vi "Image_Save_Handler_2.0.vi"(0 "first iteration":bool, 4 "Data":T1={"Camera 1"={"Camera1"="", "Cam 1"=FALSE, "CAM1 Model"=enum."a2A5328-15ucBAS", "Cam1 ID"=0}, "Camera 2"={"Camera2"="", "Cam 2"=FALSE, "CAM2 Model"=enum."a2A5328-15ucBAS", "Cam2 ID"=0}, "Image"={"Camera1_Img"=refnum, "Camera2_Img"=refnum, "Img1_Orig_Disp"=refnum, "Img2_Orig_Disp"=refnum, "Img1_Orig_RGB"=refnum, "Img2_Orig_RGB"=refnum, "Blue_Plane_Extract"=refnum, "Subtracted_Plane"=refnum, "Img1_Binary"=refnum, "Img2_Binary"=refnum, "Crop_Mask"=refnum, "Img1_Save"=refnum, "Img2_Save"=refnum, "Img1_Cali_Full"=refnum, "Img2_Cali_Full"=refnum, "Img1_Cali_Detect"=refnum, "Img2_Cali_Detect"=refnum}, "Ques"={"Cam 1 queue"=refnum, "Cam 2 queue"=refnum, "Cam 1 - save queue"=refnum, "Cam 2 - save queue"=refnum, "Image Process Queue Size"=500, "Image Save Queue Size"=500, "Overload threshold"=500, "Max large object threshold"=0}, "Arduino SRS"={"Pinch-valve"="", "Actuator"=FALSE, "Arduino Uno"="", "Valve state"=enum."Open"}, "Pump"={"Port"="", "Connection"=FALSE, "Flush Size"=0, "Command"="", "Pump Size"=enum."Large", "Pump"="", "Ready"=FALSE}, "Camera settings"={"Detection settings"={"Sample size threshold"=500, "Detection Region %"=30.0, "Timeout Sample"=200}, "Lens/camera settings"={"Aperture"=enum."Item 0", "Legacy Cam Attributes"=FALSE, "Max Framerate"=100, "Exposure Time"=1000.0, "Framerate"=15}, "Crop settings"={"Cam1"={"Rectangle 1"={"Left"=0, "Top"=0, "Right"=0, "Bottom"=0, "Rotation"=0.0}, "Camera Orientation 1"="", "Pixel to mm 1"=0.0}, "Cam2"={"Rectangle 2"={"Left"=0, "Top"=0, "Right"=0, "Bottom"=0, "Rotation"=0.0}, "Camera Orientation 2"="", "Pixel to mm 2"=0.0}}}, "Arduino ISS"={"Mega F3"="", "Phase3"=FALSE, "Barcode"="", "Sorting sys."=FALSE, "Initial size"=0.0, "Size Interval"=0.0, "Mun. of containers"=0.0, "Container nr."=0.0, "Arduino Mega"="", "Attempts"=0.0}, "Img_Capt"=FALSE, "Empty_Refill"=FALSE, "I don't think is in use"={"Light intensity"=100}, "Extended setup"={"Location"="Station", "Latitude"="Station", "Longitude"="Station", "Determiner"="Station", "Sex"="Station", "Station"="", "Collection date"=""}, "Main interface"={"Sample Name"="Test Sample", "Operator"="JFR", "Species Name"="", "Other Notes"=""}, "Tap1"=0, "SystemVersion"=0, "System Serial"="", "Exit"=FALSE, "Kuvette Full"=FALSE, "Core JKI"={"Current VI Reference"=refnum, "Close Panel on Exit?"=FALSE}, "Calibration"={"Calibration 1"=path "C:/Users/au540322/Desktop/IHS_Project/images/Debris/Debris_0/Debris_0_2019_06_01-23-32-49-686.PNG", "Calibration 2"=path "C:/Users/au540322/Desktop/IHS_Project/images/Debris/Debris_0/Debris_0_2019_06_01-23-32-49-686.PNG", "Detect 1"=path "C:/Users/au540322/Desktop/IHS_Project/images/Debris/Debris_0/Debris_0_2019_06_01-23-32-49-686.PNG", "Detect 2"=path "C:/Users/au540322/Desktop/IHS_Project/images/Debris/Debris_0/Debris_0_2019_06_01-23-32-49-686.PNG"}, "Auto Flush"=FALSE, "Status History"="", "Timestamp Start"=""} {"SystemVersion" items=["Standard", "XL"]; "Tap1" items=["Session Data", "Extended Setup", "Buffer", "Camera", "Dispenser", "Stats", "Connections"]; "I don't think is in use"."Light intensity" scale=0.0..100.0; "Camera settings"."Crop settings"."Cam2"."Rectangle 2"."Rotation" format="%.2f"; "Camera settings"."Crop settings"."Cam2"."Rectangle 2"."Left" scale=0.0..1024.0; "Camera settings"."Crop settings"."Cam2"."Rectangle 2"."Right" scale=0.0..1024.0; "Camera settings"."Crop settings"."Cam1"."Rectangle 1"."Rotation" format="%.2f"; "Camera settings"."Crop settings"."Cam1"."Rectangle 1"."Left" scale=0.0..1024.0; "Camera settings"."Crop settings"."Cam1"."Rectangle 1"."Right" scale=0.0..1024.0; "Camera settings"."Lens/camera settings"."Framerate" min=1; "Camera settings"."Lens/camera settings"."Max Framerate" min=1; "Camera settings"."Detection settings"."Sample size threshold" min=1; "Pump"."Flush Size" min=0 max=6000 step=100; "Ques"."Overload threshold" min=1; "Ques"."Image Save Queue Size" min=1; "Ques"."Image Process Queue Size" min=1}, 7 "Stop?":bool) -> (12 "Image Save 1":T3, 13 "Container num. Out":i32=2, 14 "Image Save 2":T3, 15 "Container barcode":string, 17 "Cam2_Stats":cluster{"Mean_Area":i32, "Img_Count":u32} caption="Camera 2", 18 "Ready file created":bool, 19 "Cam1_Stats":cluster{"Mean_Area":i32, "Img_Count":u32} caption="Camera 1", 20 "Queue size":T5, 23 "timeout":bool, 24 "max queue":i32, 25 "Sample Name":string, 27 "Stop out":bool)   [LabVIEW 2024]
doc: "Saves image files from cameras in specified folder location."
uses:
  <vilib>/vision/Image Controls.llb/IMAQ Image.ctl
  controls/Data_JKI.ctl
  <vilib>/userDefined/High Color/IMAQdx.ctl
  Camera_ID.ctl
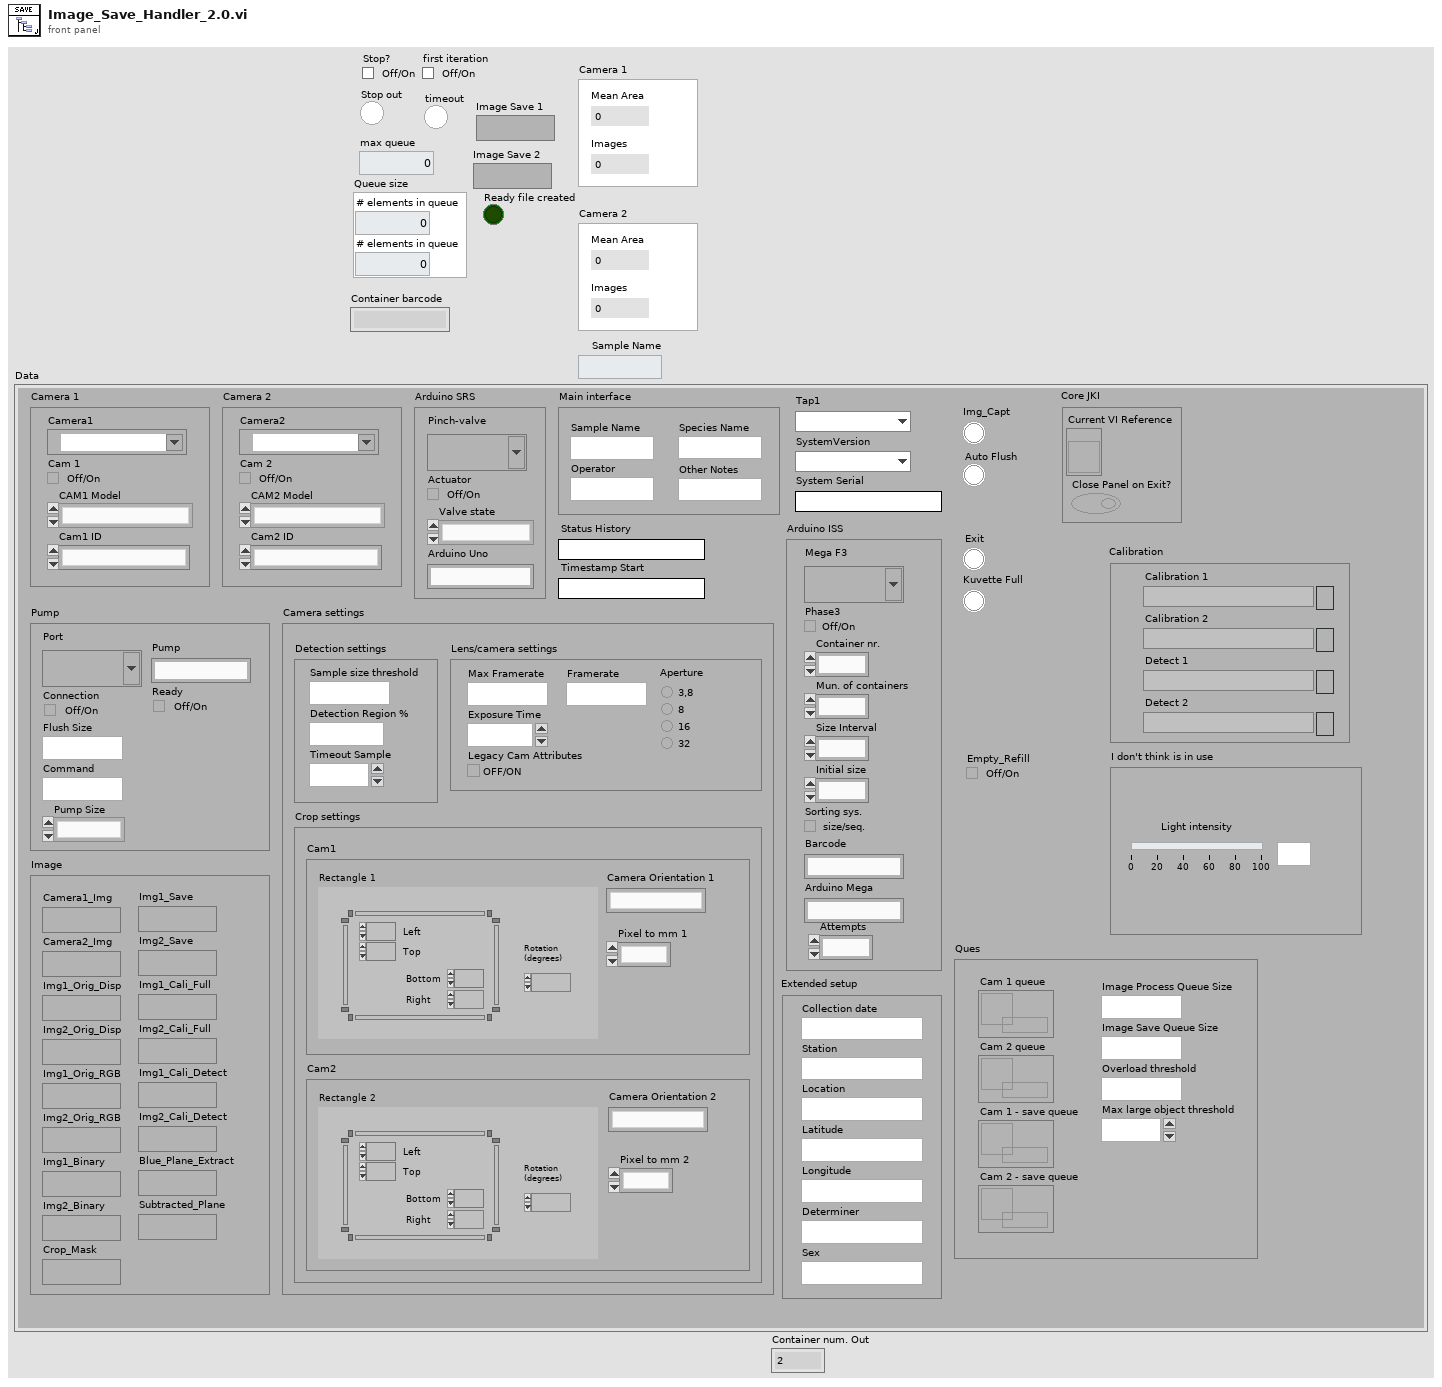
[diagram p1: front panel]
types:
  T1 = typedef "Data_JKI.ctl" = cluster{"Camera 1":cluster{"Camera1":T2, "Cam 1":bool, "CAM1 Model":enum16{"a2A5328-15ucBAS", "acA1920-155uc"}, "Cam1 ID":i32}, "Camera 2":cluster{"Camera2":T2, "Cam 2":bool, "CAM2 Model":enum16{"a2A5328-15ucBAS", "acA1920-155uc"}, "Cam2 ID":i32}, "Image":cluster{"Camera1_Img":T3, "Camera2_Img":T3, "Img1_Orig_Disp":T3, "Img2_Orig_Disp":T3, "Img1_Orig_RGB":T3, "Img2_Orig_RGB":T3, "Blue_Plane_Extract":T3, "Subtracted_Plane":T3, "Img1_Binary":T3, "Img2_Binary":T3, "Crop_Mask":T3, "Img1_Save":T3, "Img2_Save":T3, "Img1_Cali_Full":T3, "Img2_Cali_Full":T3, "Img1_Cali_Detect":T3, "Img2_Cali_Detect":T3}, "Ques":cluster{"Cam 1 queue":refnum<queue>, "Cam 2 queue":refnum<queue>, "Cam 1 - save queue":refnum<queue>, "Cam 2 - save queue":refnum<queue>, "Image Process Queue Size":i32, "Image Save Queue Size":i32, "Overload threshold":i32, "Max large object threshold":i32}, "Arduino SRS":cluster{"Pinch-valve":refnum<visa-resource-name>, "Actuator":bool, "Arduino Uno":string, "Valve state":enum16{"Standby", "Close", "Open"}}, "Pump":cluster{"Port":refnum<visa-resource-name>, "Connection":bool, "Flush Size":i32, "Command":string, "Pump Size":enum16{"None", "Small", "Large"}, "Pump":string, "Ready":bool}, "Camera settings":cluster{"Detection settings":cluster{"Sample size threshold":i32, "Detection Region %":dbl, "Timeout Sample":i32}, "Lens/camera settings":cluster{"Aperture":enum32{"Item 0", "Item 1", "Item 2", "Item 3"}, "Legacy Cam Attributes":bool, "Max Framerate":i32, "Exposure Time":dbl, "Framerate":i32}, "Crop settings":cluster{"Cam1":cluster{"Rectangle 1":T4, "Camera Orientation 1":string, "Pixel to mm 1":dbl}, "Cam2":cluster{"Rectangle 2":T4, "Camera Orientation 2":string, "Pixel to mm 2":dbl}}}, "Arduino ISS":cluster{"Mega F3":refnum<visa-resource-name>, "Phase3":bool, "Barcode":string, "Sorting sys.":bool, "Initial size":dbl, "Size Interval":dbl, "Mun. of containers":dbl, "Container nr.":dbl, "Arduino Mega":string, "Attempts":dbl}, "Img_Capt":bool, "Empty_Refill":bool, "I don't think is in use":cluster{"Light intensity":i32}, "Extended setup":cluster{"Location":string, "Latitude":string, "Longitude":string, "Determiner":string, "Sex":string, "Station":string, "Collection date":string}, "Main interface":cluster{"Sample Name":string, "Operator":string, "Species Name":string, "Other Notes":string}, "Tap1":u16, "SystemVersion":u16, "System Serial":string, "Exit":bool, "Kuvette Full":bool, "Core JKI":cluster{"Current VI Reference":refnum<vi>, "Close Panel on Exit?":bool}, "Calibration":cluster{"Calibration 1":path, "Calibration 2":path, "Detect 1":path, "Detect 2":path}, "Auto Flush":bool, "Status History":string, "Timestamp Start":string}
  T2 = typedef "IMAQdx.ctl" = refnum<k21>
  T3 = typedef "IMAQ Image.ctl" = refnum<image>
  T4 = typedef "IMAQ Rectangle" = cluster{"Left":i32, "Top":i32, "Right":i32, "Bottom":i32, "Rotation":dbl}
  T5 = cluster{"# elements in queue":i32, "# elements in queue":i32}
  T6 = typedef "Camera_ID.ctl" = enum16{"Camera 1", "Camera 2"}
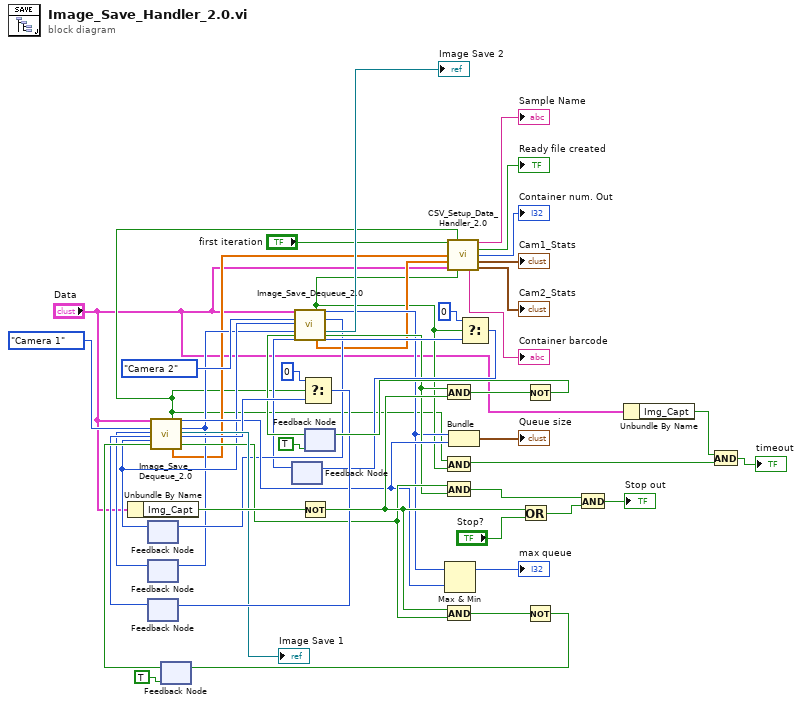
[diagram p0: block diagram]
diagram:
  n1 = Unbundle By Name("Data") -> ("Img_Capt"=w48:bool)
  n2 = feedback #1() -> (w19:i32)  [unwired: 1 in]
  n3 = feedback #2() -> (w26:i32)  [unwired: 1 in]
  n4 = feedback #3() -> (w27:u32)  [unwired: 1 in]
  n5 = feedback #4(TRUE) -> (w28:bool)
  n6 = call "Image_Save_Dequeue_2.0.vi"("Data"="Data", "Camera"=Camera_ID."Camera 1", "Old"=w26, "cam1_prev"=w27, "Other"=w19, "Queue active"=w28) -> ("timed out?"=w5:bool, "Sample Data"=w8:dbl[], "# elements in queue"=w29:i32, "State out"=w18:i32, "Image Save 1"=→"Image Save 1":T3, "cam1_count"=w30:u32, "Last image"=w31:bool)  [unwired: 13 in, 2 out]
  n7 = feedback-in #2(w18) -> ()
  n8 = feedback #5() -> (w17:u32)  [unwired: 1 in]
  n9 = Not(x=w48) -> (.not. x?=w46:bool)
  n10 = Select(t=u32 0, s=w5, f=w30) -> (s? t:f=w37:u32)
  n11 = feedback-in #3(w37) -> ()
  n12 = feedback #6(TRUE) -> (w24:bool)
  n13 = call "Image_Save_Dequeue_2.0.vi"("Data"="Data", "Camera"=Camera_ID."Camera 2", "Old"=w19, "Other"=w18, "Queue active"=w24, "cam2_prev"=w17) -> ("timed out?"=w7:bool, "Sample Data"=w9:dbl[], "# elements in queue"=w16:i32, "State out"=w20:i32, "Image Save 2"=→"Image Save 2":T3, "Last image"=w21:bool, "cam2_count"=w22:u32)  [unwired: 13 in, 2 out]
  n14 = feedback-in #1(w20) -> ()
  n15 = And(x=w21, y=w46) -> (x .and. y?=w47:bool)
  n16 = And(x=w5, y=w7) -> (x .and. y?=w1:bool)
  n17 = And(x=w31, y=w21) -> (x .and. y?=w51:bool)
  n18 = And(x=w46, y=w31) -> (x .and. y?=w45:bool)
  n19 = Max & Min(x=w16, y=w29) -> (max(x,y)=→"max queue":i32)  [unwired: 1 out]
  n20 = call "CSV_Setup_Data_Handler_2.0.vi"("first iteration"="first iteration", "Timeout 1"=w5, "Sample Data"=w8, "Sample Data 2"=w9, "Data"="Data", "Timeout 2"=w7) -> ("Sample Name"=→"Sample Name":string, "Ready file created"=→"Ready file created":bool, "Container num. Out"=→"Container num. Out":i32, "Cam1_Stats"=→"Cam1_Stats":cluster{"Mean_Area":i32, "Img_Count":u32}, "Container barcode"=→"Container barcode":string, "Cam2_Stats"=→"Cam2_Stats":cluster{"Mean_Area":i32, "Img_Count":u32})  [unwired: 4 in]
  n21 = Bundle("# elements in queue"=w16, "# elements in queue"=w29) -> (→"Queue size":T5)  [unwired: 1 in]
  n22 = Select(t=u32 0, s=w7, f=w22) -> (s? t:f=w35:u32)
  n23 = feedback-in #5(w35) -> ()
  n24 = Or(x=w46, y="Stop?") -> (x .or. y?=w49:bool)
  n25 = Not(x=w47) -> (.not. x?=w42:bool)
  n26 = feedback-in #6(w42) -> ()
  n27 = Not(x=w45) -> (.not. x?=w43:bool)
  n28 = feedback-in #4(w43) -> ()
  n29 = And(x=w51, y=w49) -> (x .and. y?=→"Stop out":bool)
  n30 = Unbundle By Name("Data") -> ("Img_Capt"=w2:bool)
  n31 = And(x=w2, y=w1) -> (x .and. y?=→"timeout":bool)
